vi "NPCC Errors.vi"(8 "error in (no error)":errorcluster, 11 "[error code] (0)":i32 format="%0.0f") -> (0 "error out":errorcluster)   [LabVIEW 2014]
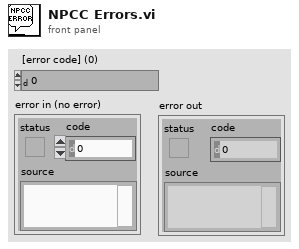
[diagram p1: front panel]
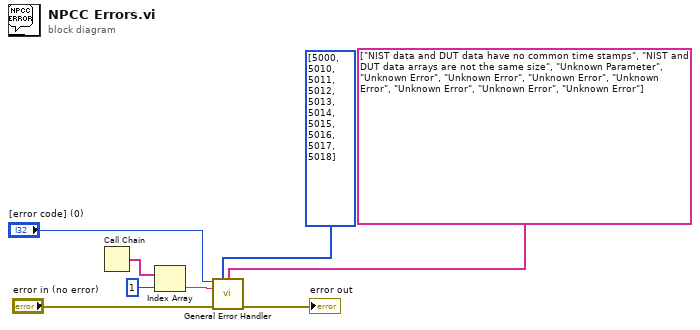
[diagram p0: block diagram]
diagram:
  n1 = Call Chain() -> (call chain=w3:string[])
  n2 = Index Array(array=w3, index=1) -> (element=w1:string)
  n3 = call <vilib>:"General Error Handler.vi"("[error code] (0)"="[error code] (0)", "[user-defined codes]"=i32[] [5000, 5010, 5011, 5012, 5013, 5014, 5015, 5016, 5017, 5018], "[user-defined descriptions]"=string[] ["NIST data and DUT data have no common time stamps", "NIST and DUT data arrays are not the same size", "Unknown Parameter", "Unknown Error", "Unknown Error", "Unknown Error", "Unknown Error", "Unknown Error", "Unknown Error", "Unknown Error"], "[error source] (\" \")"=w1, "error in (no error)"="error in (no error)") -> ("error out"=→"error out":errorcluster)  [unwired: 6 in, 4 out]
